vi "GUI.vi"() -> ()   [LabVIEW 2015]
uses:
  <vilib>/Instr/_visa.llb/VISA Configure Serial Port (Instr).vi
  <vilib>/sound2/lvsound2.llb/Sound File Write Open.vi
  <vilib>/express/express analysis/Spectral/Block/exnSpectralBlock spectral measurements power poly.vi
  <vilib>/express/express analysis/Spectral/Block/exnSpectralBlock spectral measurements power DDT.vi
  <vilib>/sound2/lvsound2.llb/Sound File Write (DBL).vi
  <vilib>/express/express analysis/Spectral/XNode/ExpressSpectralMeasurementsBlockNode.xnode
panel:
  out "Timer":dbl
  in  "Time":dbl
  in  "Amplitude Cutoff":dbl
  out "Serial String":string
  in  "Record":bool
  in  "VISA resource name":refnum<visa-resource-name>="COM1"
  in  "Upper Frequency Cut-Off":dbl=2500.0 caption="Upper Cut-Off"
  in  "Lower Frequency Cut-Off":dbl=450.0 caption="Lower Cut-Off"
  out "Time Data":dynamicdata(graph)
  out "Waveform Graph":dynamicdata(graph)=[{"t0"=timestamp(0 s since 1904-01-01), "dt"=2.666666666666669, "Y"=array[6000 elements], "attributes"=variant("NI_ChannelName"=variant(string "Left Channel (Power Spectrum)"), "NI_OriginalChannelName"=variant(string "Left Channel"), "NI_UnitDescription"=variant(string "Volts"))}, {"t0"=timestamp(0 s since 1904-01-01), "dt"=2.666666666666669, "Y"=array[6000 elements], "attributes"=variant("NI_ChannelName"=variant(string "Right Channel (Power Spectrum)"), "NI_OriginalChannelName"=variant(string "Right Channel"), "NI_UnitDescription"=variant(string "Volts"))}]
  in  "Volume":dbl(slide)=0.125 scale=0.0..100.0
  in  "Bass":dbl(slide)=0.4693877551020408 scale=0.0..5.0
  in  "Midtone":dbl(slide)=0.4081632653061224 scale=0.0..5.0
  in  "Treble":dbl(slide)=0.4081632653061224 scale=0.0..5.0
  in  "stop (F)":bool
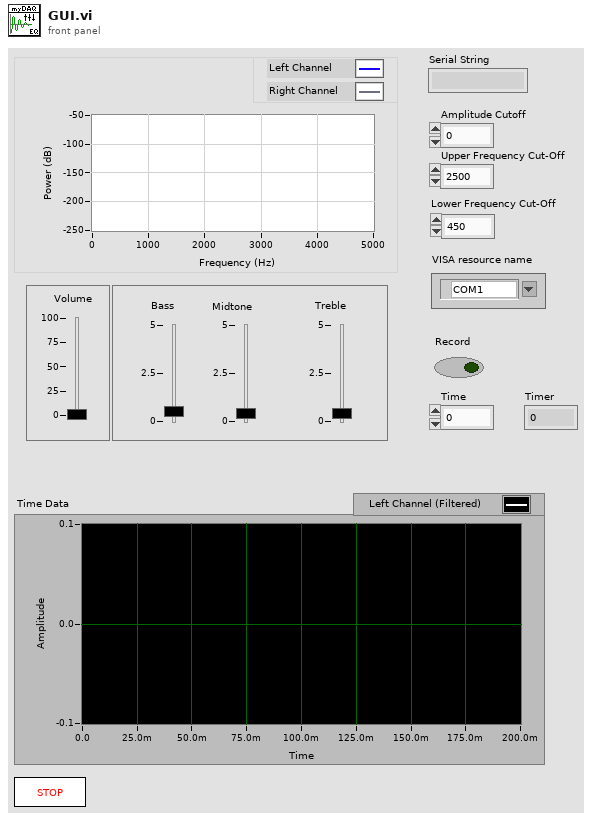
[diagram p1: front panel]
types:
  T1 = typedef "Sound File Refnum.ctl" = refnum<file>
  T2 = cluster{"averaging mode":u16, "weighting mode":u16, "number of averages":u32}
  T3 = cluster{"dB On (F)":bool, "unwrap phase (F)":bool, "convert to degree (F)":bool}
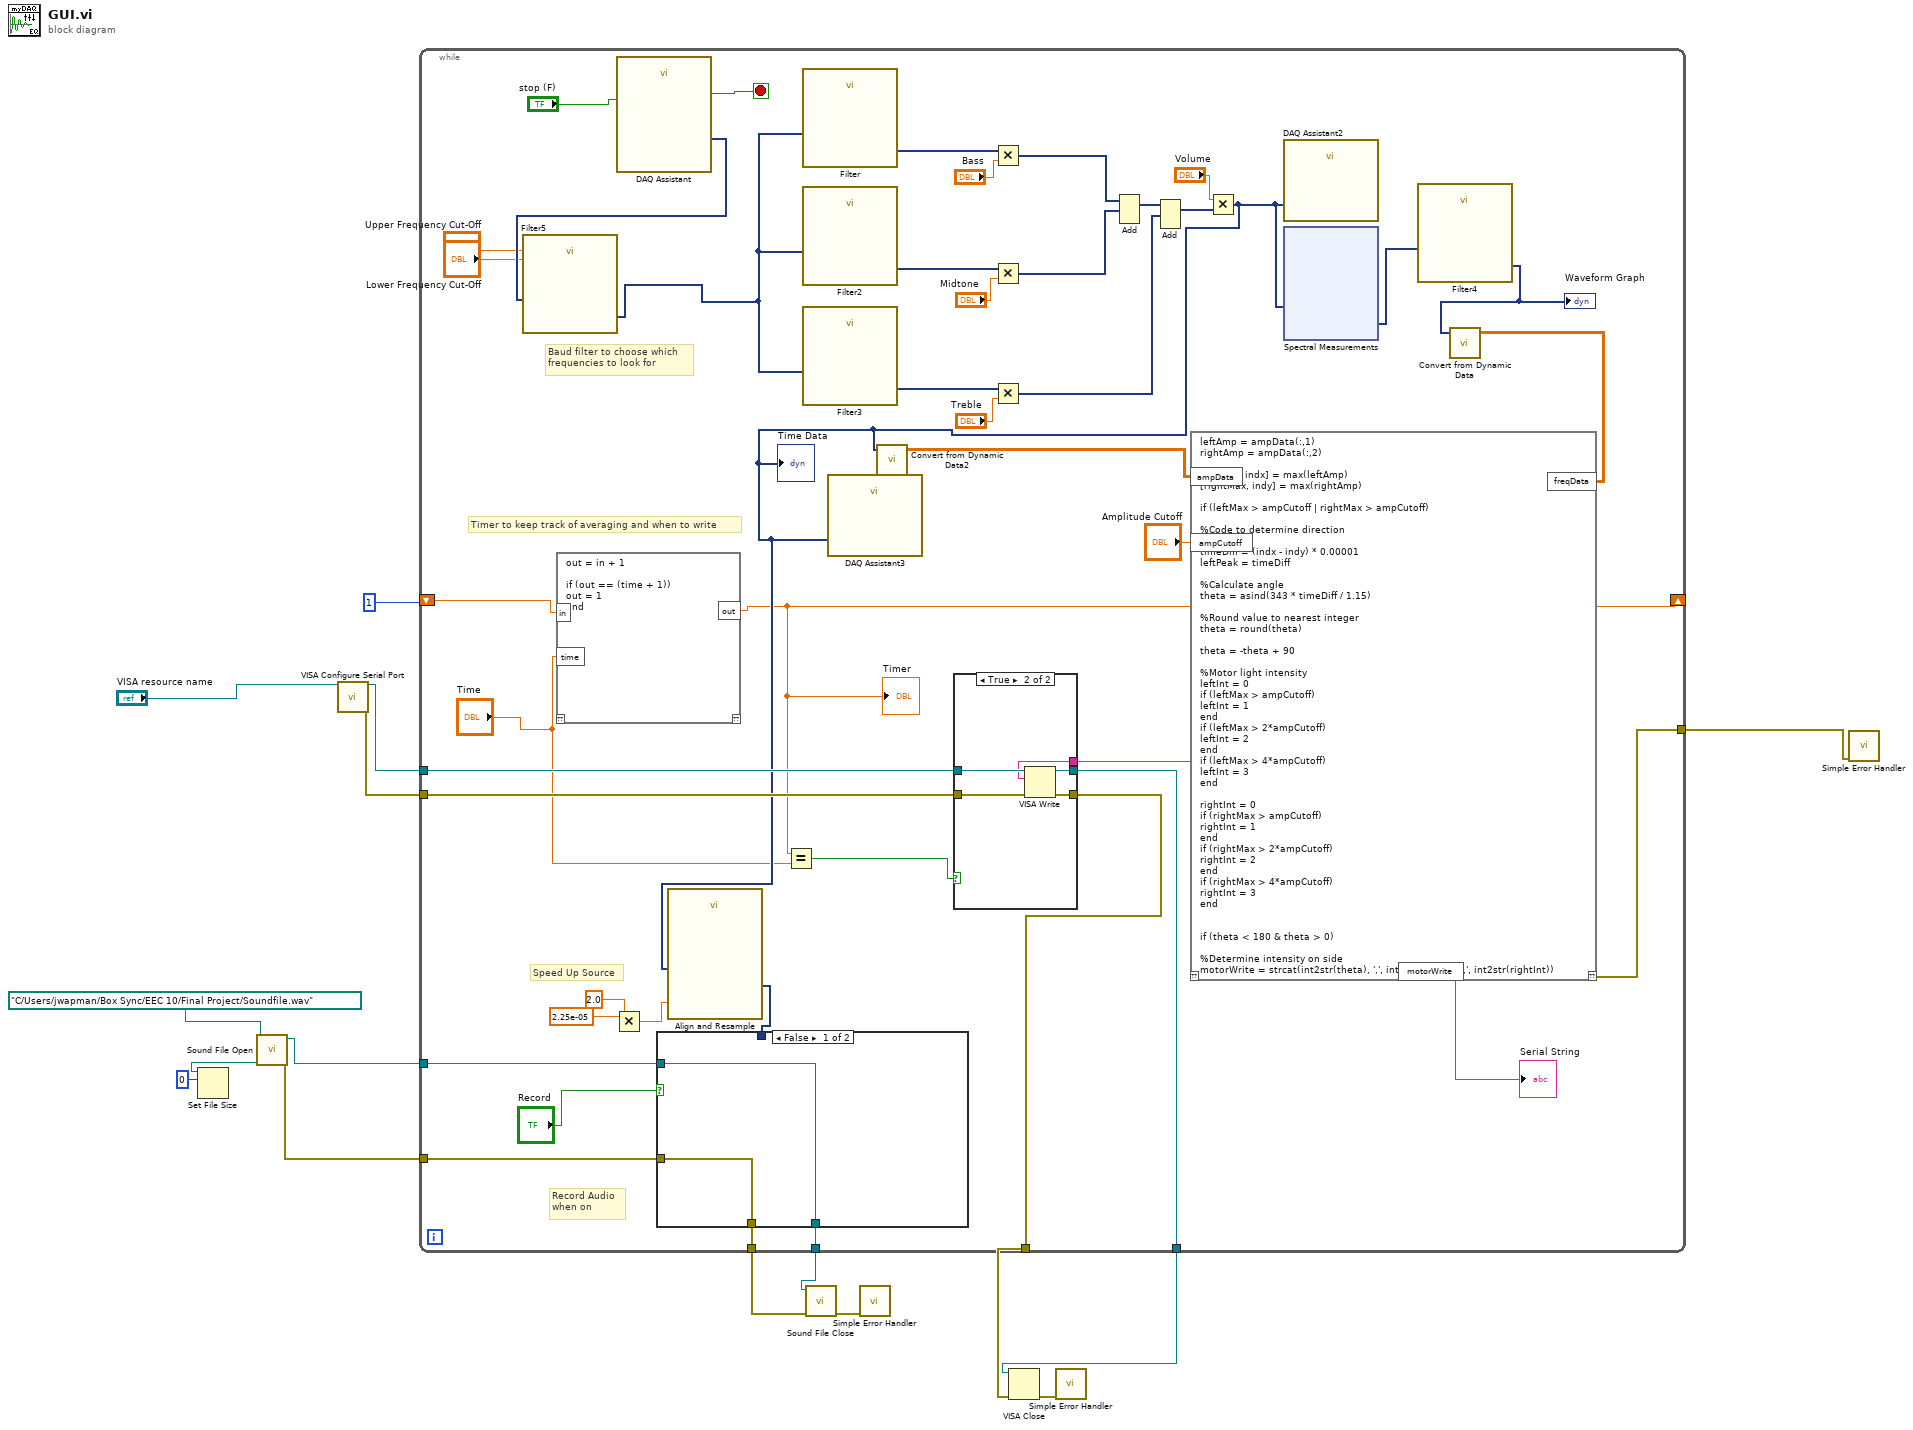
[diagram p0: block diagram]
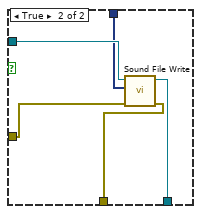
[diagram p2: hidden frame]
diagram:
  w2 = path "C:/Users/jwapman/Box Sync/EEC 10/Final Project/Soundfile.wav"
  n1 = Set File Size(6:i64 0 ("size (in bytes)"), 7:w2) -> ()  [unwired: 1 in, 2 out]
  n2 = call-poly <vilib>:"Sound File Open.vi"("path"=w2) -> ("error out"=w7:errorcluster, "sound file refnum"=w8:T1)  [unwired: 9 in]
  n3 = call-poly "VISA Configure Serial Port"("VISA resource name"="VISA resource name") -> ("VISA resource name out"=w10:refnum<visa-resource-name>, "error out"=w9:errorcluster)  [unwired: 9 in, 4 out]
  n4 = while {
    shift-right: [w16] -> _
    shift-left: 1 -> [w39]
    tunnel: [w38] -> w12
    tunnel: [w37] -> w11
    tunnel: w10 -> [w36]
    tunnel: w9 -> [w35]
    tunnel: w8 -> [w31]
    tunnel: w7 -> [w30]
    tunnel: [w29] -> w4
    tunnel: [w28] -> w5
    tunnel: [w21] -> w1
    stop <- w58 stop-if-true
    # "Record Audio\nwhen on"
    # "Speed Up Source"
    # "Baud filter to choose which\nfrequencies to look for"
    # "Timer to keep track of averaging and when to write"
    n5 = script code="out = in + 1\n\nif (out == (time + 1))\nout = 1\nend"("in"=w39, "time"="Time") -> ("out"=w16:dbl)  [unwired: 1 in, 1 out]
    "Timer" <- w16
    n6 = Multiply(x=2.25e-05, y=2.0) -> (x*y=w26:dbl)
    n7 = call "DAQ Assistant"("stop (F)"="stop (F)") -> ("data"=w42:dynamicdata, "stopped"=w58:bool)  [unwired: 15 in, 2 out]
    n8 = call "Filter5"("Lower Cut-Off"="Lower Frequency Cut-Off", "Upper Cut-Off"="Upper Frequency Cut-Off", "Signal"=w42) -> ("Filtered Signal"=w33:dynamicdata)  [unwired: 7 in, 1 out]
    n9 = Equal?(x=w16, y="Time") -> (x = y?=w34:bool)
    n10 = call "Filter"("Signal"=w33) -> ("Filtered Signal"=w54:dynamicdata)  [unwired: 9 in, 1 out]
    n11 = call "Filter2"("Signal"=w33) -> ("Filtered Signal"=w56:dynamicdata)  [unwired: 9 in, 1 out]
    n12 = call "Filter3"("Signal"=w33) -> ("Filtered Signal"=w52:dynamicdata)  [unwired: 9 in, 1 out]
    n13 = Multiply(x=w54, y="Bass") -> (x*y=w49:dynamicdata)
    n14 = Multiply(x=w56, y="Midtone") -> (x*y=w48:dynamicdata)
    n15 = Multiply(x=w52, y="Treble") -> (x*y=w50:dynamicdata)
    n16 = Add(1:w48, 2:w49) -> (0:w57:dynamicdata)  [unwired: 1 in, 1 out]
    n17 = Add(1:w50, 2:w57) -> (0:w47:dynamicdata)  [unwired: 1 in, 1 out]
    n18 = Multiply(x="Volume", y=w47) -> (x*y=w19:dynamicdata)
    "Time Data" <- w19
    n19 = call "Align and Resample"("dt"=w26, "Signals"=w19) -> ("Resampled Signals"=w25:dynamicdata)  [unwired: 7 in, 2 out]
    n20 = case shown="False" "Record" {
      tunnel: w31 -> [w59 w65]
      tunnel: w30 -> [w60 w64]
      tunnel: [w60 w63] -> w29
      tunnel: [w59 w62] -> w28
      tunnel: w25 -> [_ w61]
      frame False {
      }
      frame True {
        n21 = call-poly <vilib>:"Sound File Write.vi"("error in (no error)"=w64, "data"=w61, "sound file refnum"=w65) -> ("error out"=w63:errorcluster, "sound file refnum out"=w62:T1)  [unwired: 7 in]
      }
    }
    n22 = call "DAQ Assistant3"("data"=w19) -> ()  [unwired: 16 in, 3 out]
    n23 = call "Convert from Dynamic Data2"("Dynamic Data Type"=w19) -> ("Array"=w22:dbl[][])  [unwired: 3 in]
    n24 = call "DAQ Assistant2"("data"=w19) -> ()  [unwired: 16 in, 3 out]
    n25 = xnode "Spectral Measurements"("Signals"=w19) -> ("Power Spectrum"=w44:dynamicdata)  [unwired: 1 in, 1 out]
    n26 = call "Filter4"("Signal"=w44) -> ("Filtered Signal"=w43:dynamicdata)  [unwired: 9 in, 1 out]
    "Waveform Graph" <- w43
    n27 = call "Convert from Dynamic Data"("Dynamic Data Type"=w43) -> ("Array"=w23:dbl[][])  [unwired: 3 in]
    n28 = script code="leftAmp = ampData(:,1)\nrightAmp = ampData(:,2)\n\n[leftMax, indx] = max(leftAmp)\n[rightMax, indy] = max(rightAmp)\n\nif (leftMax > ampCutoff | rightMax > ampCutoff)\n\n%Code to determine direction\n\ntimeDiff = (indx - indy) * 0.00001\nleftPeak = timeDiff\n\n%Calculate angle\ntheta = asind(343 * timeDiff / 1.15)\n\n%Round value to nearest integer\ntheta = round(theta)\n\ntheta = -theta + 90\n\n%Motor light intensity\nleftInt = 0\nif (leftMax > ampCutoff)\nleftInt = 1\nend\nif (leftMax > 2*ampCutoff)\nleftInt = 2\nend\nif (leftMax > 4*ampCutoff)\nleftInt = 3\nend\n\nrightInt = 0\nif (rightMax > ampCutoff)\nrightInt = 1\nend\nif (rightMax > 2*ampCutoff)\nrightInt = 2\nend\nif (rightMax > 4*ampCutoff)\nrightInt = 3\nend\n\n\nif (theta < 180 & theta > 0)\n\n%Determine intensity on side\nmotorWrite = strcat(int2str(theta), ',', int2str(leftInt), ',', int2str(rightInt))\n\n\n\n\nend\n\nend"("freqData"=w23, "ampData"=w22, "ampCutoff"="Amplitude Cutoff") -> ("??"=w21:errorcluster, "motorWrite"=w20:string)  [unwired: 1 in]
    "Serial String" <- w20
    n29 = case shown="True" w34 {
      tunnel: [w67 w72] -> w38
      tunnel: [w66 w71] -> w37
      tunnel: w36 -> [w67 w70]
      tunnel: w35 -> [w66 w69]
      tunnel: w20 -> [_ w68]
      frame False {
      }
      frame True {
        n30 = VISA Write(VISA resource name=w70, write buffer=w68, error in (no error)=w69) -> (VISA resource name out=w72:refnum<visa-resource-name>, error out=w71:errorcluster)  [unwired: 1 out]
      }
    }
  }
  n31 = call <vilib>:"Sound File Close.vi"("error in (no error)"=w4, "sound file refnum"=w5) -> ("error out"=w6:errorcluster)  [unwired: 9 in]
  n32 = call <vilib>:"Simple Error Handler.vi"("error in (no error)"=w6) -> ()  [unwired: 4 in, 5 out]
  n33 = VISA Close(VISA resource name=w12, error in (no error)=w11) -> (error out=w13:errorcluster)
  n34 = call <vilib>:"Simple Error Handler.vi"("error in (no error)"=w13) -> ()  [unwired: 1 in, 8 out]
  n35 = call <vilib>:"Simple Error Handler.vi"("error in (no error)"=w1) -> ()  [unwired: 4 in, 5 out]
